vi "Lab Panel V6.00.vi"() -> ()   [LabVIEW 2017] (continued)
                  frame True {
                    n1786 = local read "DISP LAB05-1"() -> (w3328:T4)
                    n1787 = Unbundle(w3328) -> ("CYCLE"=w3336:dbl, "STATUS"=w3333:string)  [unwired: 1 out]
                    n1788 = global write "Global display 2.vi" "DISP LAB05-1"(w3328) -> ()
                    n1789 = Not Equal?(x=w3333, y="RUN") -> (x != y?=w3335:bool)
                    n1790 = local read "TDMS LAB05-1"() -> (w3339:refnum<k34>)
                    n1791 = Greater?(x=w3336, y=2.0) -> (0:w3337:bool)
                    n1792 = And(x=w3337, y=w3335) -> (x .and. y?=w3334:bool)
                    n1793 = case shown="True" w3334 {
                      tunnel: w3328 -> [_ w3347]
                      tunnel: w3339 -> [_ w3346]
                      tunnel: w3333 -> [_ w3345]
                      tunnel: w3332 -> [_ w3344]
                      tunnel: w3331 -> [_ w3343]
                      tunnel: w3330 -> [_ w3342]
                      tunnel: w3329 -> [_ w3341]
                      frame False {
                      }
                      frame True {
                        n1794 = stacked-sequence {
                          tunnel: w3347 -> [w3350 _ _]
                          tunnel: w3346 -> [_ w3352 _]
                          tunnel: w3345 -> [_ _ w3358]
                          tunnel: w3344 -> [_ _ w3357]
                          tunnel: w3343 -> [_ _ w3356]
                          tunnel: w3342 -> [_ _ w3355]
                          tunnel: w3341 -> [_ _ w3354]
                          frame #0 {
                            w3348 = FALSE
                            n1795 = local write "mail control"("END") -> ()
                            n1796 = Bundle(cluster=w3350) -> (w3351:T4)  [unwired: 3 in]
                            n1797 = local write "O/I  LAB05-1"(w3348) -> ()
                            n1798 = local write "RUN LAB05-1"(w3348) -> ()
                            n1799 = local write "run lab05-1"(w3348) -> ()
                            n1800 = local write "DISP LAB05-1"(w3351) -> ()
                          }
                          frame #1 {
                            n1801 = TDMS Close(11:w3352) -> (0:w3353:errorcluster)  [unwired: 1 in, 1 out]
                            n1802 = local write "data file error"(w3353) -> ()
                          }
                          frame #2 {
                            n1803 = stacked-sequence {
                              tunnel: "LAB05-1" -> [w3361 w3367]
                              tunnel: w3358 -> [_ w3366]
                              tunnel: w3357 -> [_ w3365]
                              tunnel: w3356 -> [_ w3364]
                              tunnel: w3355 -> [_ w3363]
                              tunnel: w3354 -> [_ w3362]
                              frame #0 {
                                n1804 = call "sub vi - defrag tdms v1.vi"("panel id"=w3361) -> ("error out"=w3360:errorcluster)  [unwired: 10 in]
                                n1805 = local write "data file error"(w3360) -> ()
                              }
                              frame #1 {
                                n1806 = Bundle("STATUS"=w3366, "OUT SERVER ADDRESS"=w3365, "FROM ACCOUNT"=w3364, "Mail Test File To:"=w3363, "Mail Test Fail"=w3362) -> (w3369:T30)  [unwired: 1 in]
                                n1807 = call "Save data file (pass-fail) v5.vi"("Input Cluster"=w3369, "panel id"=w3367) -> ("network file save error"=w3368:errorcluster)  [unwired: 8 in, 1 out]
                                n1808 = local write "data file error"(w3368) -> ()
                              }
                            }
                          }
                        }
                      }
                    }
                  }
                }
              }
              frame #9 {
                # "LAB05-2"
                n1809 = local read "run lab05-2"() -> (w3374:bool)
                n1810 = case shown="True" w3374 {
                  tunnel: w3373 -> [_ w3379]
                  tunnel: w3372 -> [_ w3378]
                  tunnel: w3371 -> [_ w3377]
                  tunnel: w3370 -> [_ w3376]
                  frame False {
                  }
                  frame True {
                    n1811 = local read "DISP LAB05-2"() -> (w3375:T4)
                    n1812 = Unbundle(w3375) -> ("CYCLE"=w3383:dbl, "STATUS"=w3380:string)  [unwired: 1 out]
                    n1813 = global write "Global display 2.vi" "DISP LAB05-2"(w3375) -> ()
                    n1814 = Not Equal?(x=w3380, y="RUN") -> (x != y?=w3382:bool)
                    n1815 = local read "TDMS LAB05-2"() -> (w3386:refnum<k34>)
                    n1816 = Greater?(x=w3383, y=2.0) -> (0:w3384:bool)
                    n1817 = And(x=w3384, y=w3382) -> (x .and. y?=w3381:bool)
                    n1818 = case shown="True" w3381 {
                      tunnel: w3375 -> [_ w3394]
                      tunnel: w3386 -> [_ w3393]
                      tunnel: w3380 -> [_ w3392]
                      tunnel: w3379 -> [_ w3391]
                      tunnel: w3378 -> [_ w3390]
                      tunnel: w3377 -> [_ w3389]
                      tunnel: w3376 -> [_ w3388]
                      frame False {
                      }
                      frame True {
                        n1819 = stacked-sequence {
                          tunnel: w3394 -> [w3397 _ _]
                          tunnel: w3393 -> [_ w3399 _]
                          tunnel: w3392 -> [_ _ w3405]
                          tunnel: w3391 -> [_ _ w3404]
                          tunnel: w3390 -> [_ _ w3403]
                          tunnel: w3389 -> [_ _ w3402]
                          tunnel: w3388 -> [_ _ w3401]
                          frame #0 {
                            w3395 = FALSE
                            n1820 = local write "mail control"("END") -> ()
                            n1821 = Bundle(cluster=w3397) -> (w3398:T4)  [unwired: 3 in]
                            n1822 = local write "RUN LAB05-2"(w3395) -> ()
                            n1823 = local write "O/I  LAB05-2"(w3395) -> ()
                            n1824 = local write "run lab05-2"(w3395) -> ()
                            n1825 = local write "DISP LAB05-2"(w3398) -> ()
                          }
                          frame #1 {
                            n1826 = TDMS Close(11:w3399) -> (0:w3400:errorcluster)  [unwired: 1 in, 1 out]
                            n1827 = local write "data file error"(w3400) -> ()
                          }
                          frame #2 {
                            n1828 = stacked-sequence {
                              tunnel: "LAB05-2" -> [w3408 w3414]
                              tunnel: w3405 -> [_ w3413]
                              tunnel: w3404 -> [_ w3412]
                              tunnel: w3403 -> [_ w3411]
                              tunnel: w3402 -> [_ w3410]
                              tunnel: w3401 -> [_ w3409]
                              frame #0 {
                                n1829 = call "sub vi - defrag tdms v1.vi"("panel id"=w3408) -> ("error out"=w3407:errorcluster)  [unwired: 10 in]
                                n1830 = local write "data file error"(w3407) -> ()
                              }
                              frame #1 {
                                n1831 = Bundle("STATUS"=w3413, "OUT SERVER ADDRESS"=w3412, "FROM ACCOUNT"=w3411, "Mail Test File To:"=w3410, "Mail Test Fail"=w3409) -> (w3416:T30)  [unwired: 1 in]
                                n1832 = call "Save data file (pass-fail) v5.vi"("Input Cluster"=w3416, "panel id"=w3414) -> ("network file save error"=w3415:errorcluster)  [unwired: 8 in, 1 out]
                                n1833 = local write "data file error"(w3415) -> ()
                              }
                            }
                          }
                        }
                      }
                    }
                  }
                }
              }
            }
            n1834 = global write "Global display 2.vi" "Mail test file to:"(w2923) -> ()
            n1835 = local read "Network Directory"() -> (w2929:path)
            n1836 = global write "Global 1.vi" "Network Drive"(w2929) -> ()
          }
          frame #8 {
            # "disable functions"
            n1837 = stacked-sequence {
              tunnel: w3426 -> [w3440 _ w3497]
              tunnel: w3425 -> [w3435 _ w3496]
              tunnel: w3424 -> [w3434 _ w3495]
              tunnel: w3423 -> [w3432 _ w3494]
              tunnel: w3422 -> [w3433 _ w3493]
              tunnel: w3421 -> [_ w3457 w3492]
              tunnel: w3420 -> [_ w3458 w3491]
              tunnel: w3419 -> [_ w3459 w3490]
              tunnel: w3418 -> [_ w3460 w3489]
              tunnel: w3417 -> [_ w3461 w3488]
              frame #0 {
                n1838 = Select(t=2, s=w3432, f=0) -> (s? t:f=w3428:i32)
                n1839 = Select(t=2, s=w3434, f=0) -> (s? t:f=w3429:i32)
                n1840 = Select(t=2, s=w3433, f=0) -> (s? t:f=w3427:i32)
                n1841 = Select(t=2, s=w3440, f=0) -> (s? t:f=w3431:i32)
                n1842 = Select(t=2, s=w3435, f=0) -> (s? t:f=w3430:i32)
                n1843 = property on="SELECT LAB02-2" class="RadioBtnsControl (strict)"("DisabledEnum"=w3428) -> ()  [unwired: 2 in, 2 out]
                n1844 = property on="SELECT LAB02-1" class="RadioBtnsControl (strict)"("DisabledEnum"=w3429) -> ()  [unwired: 2 in, 2 out]
                n1845 = property on="SELECT LAB03-1" class="RadioBtnsControl (strict)"("DisabledEnum"=w3427) -> ()  [unwired: 2 in, 2 out]
                n1846 = property on="SELECT LAB01-1" class="RadioBtnsControl (strict)"("DisabledEnum"=w3431) -> ()  [unwired: 2 in, 2 out]
                n1847 = property on="SELECT LAB01-2" class="RadioBtnsControl (strict)"("DisabledEnum"=w3430) -> ()  [unwired: 2 in, 2 out]
                n1848 = Not(x=w3440) -> (.not. x?=w3441:bool)
                n1849 = property on="RESULT LAB01-1" class="Bool (strict)"("Visible"=w3441) -> ()  [unwired: 2 in, 2 out]
                n1850 = Not(x=w3435) -> (.not. x?=w3439:bool)
                n1851 = Not(x=w3434) -> (.not. x?=w3438:bool)
                n1852 = Not(x=w3432) -> (.not. x?=w3437:bool)
                n1853 = property on="RESULT LAB01-2" class="Bool (strict)"("Visible"=w3439) -> ()  [unwired: 2 in, 2 out]
                n1854 = Not(x=w3433) -> (.not. x?=w3436:bool)
                n1855 = property on="RESULT LAB02-1" class="Bool (strict)"("Visible"=w3438) -> ()  [unwired: 2 in, 2 out]
                n1856 = property on="RESULT LAB02-2" class="Bool (strict)"("Visible"=w3437) -> ()  [unwired: 2 in, 2 out]
                n1857 = property on="RESULT LAB03-1" class="Bool (strict)"("Visible"=w3436) -> ()  [unwired: 2 in, 2 out]
                n1858 = property on="SET LAB01-1" class="Clust (strict)"("DisabledEnum"=w3431) -> ()  [unwired: 2 in, 2 out]
                n1859 = property on="SET LAB01-2" class="Clust (strict)"("DisabledEnum"=w3430) -> ()  [unwired: 2 in, 2 out]
                n1860 = property on="SET LAB02-1" class="Clust (strict)"("DisabledEnum"=w3429) -> ()  [unwired: 2 in, 2 out]
                n1861 = property on="SET LAB02-2" class="Clust (strict)"("DisabledEnum"=w3428) -> ()  [unwired: 2 in, 2 out]
                n1862 = property on="SET LAB03-1" class="Clust (strict)"("DisabledEnum"=w3427) -> ()  [unwired: 2 in, 2 out]
                n1863 = property on="O/I  LAB01-1" class="Bool (strict)"("DisabledEnum"=w3431) -> ()  [unwired: 2 in, 2 out]
                n1864 = property on="O/I  LAB01-2" class="Bool (strict)"("DisabledEnum"=w3430) -> ()  [unwired: 2 in, 2 out]
                n1865 = property on="O/I  LAB02-1" class="Bool (strict)"("DisabledEnum"=w3429) -> ()  [unwired: 2 in, 2 out]
                n1866 = property on="O/I  LAB02-2" class="Bool (strict)"("DisabledEnum"=w3428) -> ()  [unwired: 2 in, 2 out]
                n1867 = property on="O/I  LAB03-1" class="Bool (strict)"("DisabledEnum"=w3427) -> ()  [unwired: 2 in, 2 out]
              }
              frame #1 {
                n1868 = Select(t=2, s=w3461, f=0) -> (s? t:f=w3452:i32)
                n1869 = Select(t=2, s=w3460, f=0) -> (s? t:f=w3453:i32)
                n1870 = Select(t=2, s=w3457, f=0) -> (s? t:f=w3456:i32)
                n1871 = Select(t=2, s=w3458, f=0) -> (s? t:f=w3455:i32)
                n1872 = Select(t=2, s=w3459, f=0) -> (s? t:f=w3454:i32)
                n1873 = property on="SELECT LAB05-2" class="RadioBtnsControl (strict)"("DisabledEnum"=w3452) -> ()  [unwired: 2 in, 2 out]
                n1874 = property on="SELECT LAB05-1" class="RadioBtnsControl (strict)"("DisabledEnum"=w3453) -> ()  [unwired: 2 in, 2 out]
                n1875 = property on="SELECT LAB03-2" class="RadioBtnsControl (strict)"("DisabledEnum"=w3456) -> ()  [unwired: 2 in, 2 out]
                n1876 = property on="SELECT LAB04-1" class="RadioBtnsControl (strict)"("DisabledEnum"=w3455) -> ()  [unwired: 2 in, 2 out]
                n1877 = property on="SELECT LAB04-2" class="RadioBtnsControl (strict)"("DisabledEnum"=w3454) -> ()  [unwired: 2 in, 2 out]
                n1878 = property on="SET LAB05-2" class="Clust (strict)"("DisabledEnum"=w3452) -> ()  [unwired: 2 in, 2 out]
                n1879 = property on="SET LAB05-1" class="Clust (strict)"("DisabledEnum"=w3453) -> ()  [unwired: 2 in, 2 out]
                n1880 = property on="SET LAB03-2" class="Clust (strict)"("DisabledEnum"=w3456) -> ()  [unwired: 2 in, 2 out]
                n1881 = property on="SET LAB04-1" class="Clust (strict)"("DisabledEnum"=w3455) -> ()  [unwired: 2 in, 2 out]
                n1882 = property on="SET LAB04-2" class="Clust (strict)"("DisabledEnum"=w3454) -> ()  [unwired: 2 in, 2 out]
                n1883 = property on="O/I  LAB05-2" class="Bool (strict)"("DisabledEnum"=w3452) -> ()  [unwired: 2 in, 2 out]
                n1884 = property on="O/I  LAB05-1" class="Bool (strict)"("DisabledEnum"=w3453) -> ()  [unwired: 2 in, 2 out]
                n1885 = property on="O/I  LAB04-1" class="Bool (strict)"("DisabledEnum"=w3455) -> ()  [unwired: 2 in, 2 out]
                n1886 = property on="O/I  LAB04-2" class="Bool (strict)"("DisabledEnum"=w3454) -> ()  [unwired: 2 in, 2 out]
                n1887 = property on="O/I  LAB03-2" class="Bool (strict)"("DisabledEnum"=w3456) -> ()  [unwired: 2 in, 2 out]
                n1888 = Not(x=w3461) -> (.not. x?=w3462:bool)
                n1889 = Not(x=w3460) -> (.not. x?=w3463:bool)
                n1890 = Not(x=w3459) -> (.not. x?=w3464:bool)
                n1891 = property on="RESULT LAB05-2" class="Bool (strict)"("Visible"=w3462) -> ()  [unwired: 2 in, 2 out]
                n1892 = property on="RESULT LAB05-1" class="Bool (strict)"("Visible"=w3463) -> ()  [unwired: 2 in, 2 out]
                n1893 = Not(x=w3458) -> (.not. x?=w3465:bool)
                n1894 = property on="RESULT LAB04-2" class="Bool (strict)"("Visible"=w3464) -> ()  [unwired: 2 in, 2 out]
                n1895 = Not(x=w3457) -> (.not. x?=w3466:bool)
                n1896 = property on="RESULT LAB04-1" class="Bool (strict)"("Visible"=w3465) -> ()  [unwired: 2 in, 2 out]
                n1897 = property on="RESULT LAB03-2" class="Bool (strict)"("Visible"=w3466) -> ()  [unwired: 2 in, 2 out]
              }
              frame #2 {
                # "disable calibrate if any test running"
                n1898 = Or(x=w3489, y=w3488) -> (x .or. y?=w3482:bool)
                n1899 = Or(x=w3491, y=w3490) -> (x .or. y?=w3484:bool)
                n1900 = Or(x=w3495, y=w3494) -> (x .or. y?=w3486:bool)
                n1901 = Or(x=w3493, y=w3492) -> (x .or. y?=w3485:bool)
                n1902 = Or(x=w3497, y=w3496) -> (x .or. y?=w3487:bool)
                n1903 = Or(x=w3485, y=w3484) -> (x .or. y?=w3483:bool)
                n1904 = Or(x=w3487, y=w3486) -> (x .or. y?=w3481:bool)
                n1905 = Or(x=w3483, y=w3482) -> (x .or. y?=w3480:bool)
                n1906 = Or(x=w3481, y=w3480) -> (x .or. y?=w3477:bool)
                "Any Test Running" <- w3477
                n1907 = case shown="False" w3477 {
                  tunnel: [0 2] -> w3479
                  frame False {
                  }
                  frame True {
                  }
                }
                n1908 = property on="JIG TEST" class="Clust (strict)"("DisabledEnum"=w3479) -> ()  [unwired: 2 in, 2 out]
                n1909 = property on="Network Directory" class="Path"("DisabledEnum"=w3479) -> ()  [unwired: 2 in, 2 out]
                n1910 = property on="MAIL SETTINGS" class="Clust (strict)"("DisabledEnum"=w3479) -> ()  [unwired: 2 in, 2 out]
                n1911 = property on="SET (cal)" class="Bool (strict)"("DisabledEnum"=w3479) -> ()  [unwired: 2 in, 2 out]
                n1912 = property on="ADMIN" class="Bool (strict)"("DisabledEnum"=0) -> ()  [unwired: 2 in, 2 out]
              }
            }
          }
          frame #9 {
            # "Note : JIG LAB0X-N   are written to digital I/O in frame 11"
            # "Drive jigs"
            n1913 = stacked-sequence {
              frame #0 {
                # "jig on"
                n1914 = local read "jig cycle"() -> (w3505:dbl)
                n1915 = property on="JIG TEST" class="Clust (strict)"() -> ("DisabledEnum"=w3502:T17)  [unwired: 2 in, 2 out]
                n1916 = Equal?(x=w3502, y=2) -> (x = y?=w3501:bool)
                n1917 = Equal?(x=w3505, y=0) -> (x = y?=w3503:bool)
                n1918 = And(x=w3503, y=w3501) -> (x .and. y?=w3500:bool)
                n1919 = case shown="True" w3500 {
                  frame False {
                  }
                  frame True {
                    n1920 = local read "run lab01-2"() -> (w3515:bool)
                    n1921 = local read "run lab01-1"() -> (w3516:bool)
                    n1922 = local read "run lab02-1"() -> (w3514:bool)
                    n1923 = local read "run lab02-2"() -> (w3513:bool)
                    n1924 = local read "run lab03-1"() -> (w3512:bool)
                    n1925 = local read "run lab03-2"() -> (w3511:bool)
                    n1926 = local read "run lab04-1"() -> (w3510:bool)
                    n1927 = local read "run lab04-2"() -> (w3509:bool)
                    n1928 = local read "run lab05-1"() -> (w3508:bool)
                    n1929 = local read "run lab05-2"() -> (w3507:bool)
                    n1930 = local write "JIG LAB01-2"(w3515) -> ()
                    n1931 = local write "JIG LAB03-2"(w3511) -> ()
                    n1932 = local write "JIG LAB01-1"(w3516) -> ()
                    n1933 = local write "JIG LAB02-1"(w3514) -> ()
                    n1934 = local write "JIG LAB02-2"(w3513) -> ()
                    n1935 = local write "JIG LAB03-1"(w3512) -> ()
                    n1936 = local write "JIG LAB04-1"(w3510) -> ()
                    n1937 = local write "JIG LAB04-2"(w3509) -> ()
                    n1938 = local write "JIG LAB05-1"(w3508) -> ()
                    n1939 = local write "JIG LAB05-2"(w3507) -> ()
                  }
                }
              }
              frame #1 {
                # "jig off"
                n1940 = local read "jig cycle"() -> (w3523:dbl)
                n1941 = local read "on loops"() -> (w3522:dbl)
                n1942 = property on="JIG TEST" class="Clust (strict)"() -> ("DisabledEnum"=w3521:T17)  [unwired: 2 in, 2 out]
                n1943 = Equal?(x=w3521, y=2) -> (x = y?=w3519:bool)
                n1944 = Equal?(x=w3523, y=w3522) -> (x = y?=w3518:bool)
                n1945 = And(x=w3518, y=w3519) -> (x .and. y?=w3517:bool)
                n1946 = case shown="True" w3517 {
                  frame False {
                  }
                  frame True {
                    w3574 = FALSE
                    w3575 = TRUE
                    w3573 = 2
                    n1947 = local read "SELECT LAB05-2"() -> (w3564:T3)
                    n1948 = local read "SELECT LAB04-2"() -> (w3566:T3)
                    n1949 = local read "SELECT LAB04-1"() -> (w3567:T3)
                    n1950 = local read "SELECT LAB05-1"() -> (w3565:T3)
                    n1951 = local read "SELECT LAB03-2"() -> (w3568:T3)
                    n1952 = local read "SELECT LAB02-1"() -> (w3571:T3)
                    n1953 = local read "SELECT LAB03-1"() -> (w3569:T3)
                    n1954 = local read "SELECT LAB02-2"() -> (w3570:T3)
                    n1955 = local read "SELECT LAB01-2"() -> (w3572:T3)
                    n1956 = local read "run lab05-1"() -> (w3534:bool)
                    n1957 = local read "run lab05-2"() -> (w3533:bool)
                    n1958 = local read "run lab04-2"() -> (w3535:bool)
                    n1959 = local read "SELECT LAB01-1"() -> (w3576:T3)
                    n1960 = local read "run lab04-1"() -> (w3536:bool)
                    n1961 = local read "run lab01-1"() -> (w3552:bool)
                    n1962 = local read "run lab01-2"() -> (w3541:bool)
                    n1963 = local read "run lab03-2"() -> (w3537:bool)
                    n1964 = local read "run lab03-1"() -> (w3538:bool)
                    n1965 = local read "run lab02-1"() -> (w3540:bool)
                    n1966 = local read "run lab02-2"() -> (w3539:bool)
                    n1967 = Equal?(x=w3573, y=w3569) -> (x = y?=w3547:bool)
                    n1968 = Equal?(x=w3573, y=w3568) -> (x = y?=w3546:bool)
                    n1969 = Equal?(x=w3573, y=w3567) -> (x = y?=w3545:bool)
                    n1970 = Equal?(x=w3573, y=w3566) -> (x = y?=w3544:bool)
                    n1971 = Equal?(x=w3573, y=w3565) -> (x = y?=w3543:bool)
                    n1972 = Equal?(x=w3573, y=w3564) -> (x = y?=w3542:bool)
                    n1973 = Equal?(x=w3573, y=w3576) -> (x = y?=w3553:bool)
                    n1974 = Equal?(x=w3573, y=w3571) -> (x = y?=w3549:bool)
                    n1975 = Equal?(x=w3573, y=w3570) -> (x = y?=w3548:bool)
                    n1976 = Equal?(x=w3573, y=w3572) -> (x = y?=w3550:bool)
                    n1977 = And(x=w3544, y=w3535) -> (x .and. y?=w3526:bool)
                    n1978 = And(x=w3547, y=w3538) -> (x .and. y?=w3529:bool)
                    n1979 = And(x=w3545, y=w3536) -> (x .and. y?=w3527:bool)
                    n1980 = And(x=w3542, y=w3533) -> (x .and. y?=w3524:bool)
                    n1981 = And(x=w3548, y=w3539) -> (x .and. y?=w3530:bool)
                    n1982 = And(x=w3546, y=w3537) -> (x .and. y?=w3528:bool)
                    n1983 = And(x=w3543, y=w3534) -> (x .and. y?=w3525:bool)
                    n1984 = And(x=w3550, y=w3541) -> (x .and. y?=w3532:bool)
                    n1985 = And(x=w3553, y=w3552) -> (x .and. y?=w3551:bool)
                    n1986 = And(x=w3549, y=w3540) -> (x .and. y?=w3531:bool)
                    n1987 = Select(t=w3575, s=w3551, f=w3574) -> (s? t:f=w3554:bool)
                    n1988 = Select(t=w3575, s=w3532, f=w3574) -> (s? t:f=w3555:bool)
                    n1989 = Select(t=w3575, s=w3531, f=w3574) -> (s? t:f=w3556:bool)
                    n1990 = Select(t=w3575, s=w3530, f=w3574) -> (s? t:f=w3557:bool)
                    n1991 = Select(t=w3575, s=w3529, f=w3574) -> (s? t:f=w3558:bool)
                    n1992 = Select(t=w3575, s=w3528, f=w3574) -> (s? t:f=w3559:bool)
                    n1993 = Select(t=w3575, s=w3527, f=w3574) -> (s? t:f=w3560:bool)
                    n1994 = Select(t=w3575, s=w3526, f=w3574) -> (s? t:f=w3561:bool)
                    n1995 = Select(t=w3575, s=w3525, f=w3574) -> (s? t:f=w3562:bool)
                    n1996 = Select(t=w3575, s=w3524, f=w3574) -> (s? t:f=w3563:bool)
                    n1997 = local write "JIG LAB03-2"(w3559) -> ()
                    n1998 = local write "JIG LAB02-1"(w3556) -> ()
                    n1999 = local write "JIG LAB02-2"(w3557) -> ()
                    n2000 = local write "JIG LAB01-2"(w3555) -> ()
                    n2001 = local write "JIG LAB03-1"(w3558) -> ()
                    n2002 = local write "JIG LAB01-1"(w3554) -> ()
                    n2003 = local write "JIG LAB05-2"(w3563) -> ()
                    n2004 = local write "JIG LAB04-1"(w3560) -> ()
                    n2005 = local write "JIG LAB05-1"(w3562) -> ()
                    n2006 = local write "JIG LAB04-2"(w3561) -> ()
                  }
                }
              }
            }
          }
          frame #10 {
            # "Note : JIG LAB0X-N   are written to digital I/O in frame 11"
            # "enable  jig test output if no test busy"
            n2007 = property on="JIG TEST" class="Clust (strict)"() -> ("DisabledEnum"=w3579:T17)  [unwired: 2 in, 2 out]
            n2008 = Equal?(x=w3579, y=0) -> (x = y?=w3577:bool)
            n2009 = case shown="True" w3577 {
              frame False {
              }
              frame True {
                n2010 = local read "JIG TEST"() -> (w3590:T11)
                n2011 = Unbundle(w3590) -> ("LAB01-1"=w3589:bool, "LAB01-2"=w3588:bool, "LAB02-1"=w3587:bool, "LAB02-2"=w3586:bool, "LAB03-1"=w3585:bool, "LAB03-2"=w3584:bool, "LAB04-1"=w3583:bool, "LAB04-2"=w3582:bool, "LAB05-1"=w3581:bool, "LAB05-2"=w3580:bool)
                n2012 = local write "JIG LAB05-1"(w3581) -> ()
                n2013 = local write "JIG LAB05-2"(w3580) -> ()
                n2014 = local write "JIG LAB04-1"(w3583) -> ()
                n2015 = local write "JIG LAB04-2"(w3582) -> ()
                n2016 = local write "JIG LAB03-2"(w3584) -> ()
                n2017 = local write "JIG LAB01-1"(w3589) -> ()
                n2018 = local write "JIG LAB02-1"(w3587) -> ()
                n2019 = local write "JIG LAB03-1"(w3585) -> ()
                n2020 = local write "JIG LAB01-2"(w3588) -> ()
                n2021 = local write "JIG LAB02-2"(w3586) -> ()
              }
            }
          }
          frame #11 {
            w3592 = FALSE
            # "Drive digital output and RESET  USB and temperature network if required."
            n2022 = global read "Global display 3.vi" "cycle O/F"() -> (w3601:bool)
            n2023 = case shown="False" w3601 {
              tunnel: [w3740 FALSE] -> w3600
              frame False {
                n2024 = local read "Analog error"() -> (w3742:bool)
                n2025 = local read "Reset Measuring"() -> (w3741:bool)
                n2026 = Or(x=w3741, y=w3742) -> (x .or. y?=w3740:bool)
              }
              frame True {
              }
            }
            n2027 = local read "O/I  LAB01-1"() -> (w3620:bool)
            n2028 = local read "JIG LAB01-1"() -> (w3619:bool)
            n2029 = local read "O/I  LAB01-2"() -> (w3618:bool)
            n2030 = local read "JIG LAB01-2"() -> (w3617:bool)
            n2031 = local read "O/I  LAB02-1"() -> (w3616:bool)
            n2032 = local read "JIG LAB02-1"() -> (w3615:bool)
            n2033 = local read "O/I  LAB02-2"() -> (w3614:bool)
            n2034 = local read "JIG LAB02-2"() -> (w3613:bool)
            n2035 = local read "O/I  LAB03-1"() -> (w3612:bool)
            n2036 = local read "JIG LAB03-1"() -> (w3611:bool)
            n2037 = local read "O/I  LAB03-2"() -> (w3610:bool)
            n2038 = local read "JIG LAB03-2"() -> (w3609:bool)
            n2039 = local read "O/I  LAB04-1"() -> (w3608:bool)
            n2040 = local read "JIG LAB04-1"() -> (w3607:bool)
            n2041 = local read "O/I  LAB04-2"() -> (w3598:bool)
            n2042 = local read "JIG LAB04-2"() -> (w3597:bool)
            n2043 = local read "O/I  LAB05-1"() -> (w3596:bool)
            n2044 = local read "JIG LAB05-1"() -> (w3595:bool)
            n2045 = local read "O/I  LAB05-2"() -> (w3594:bool)
            n2046 = local read "JIG LAB05-2"() -> (w3593:bool)
            n2047 = Build Array(w3613, w3612, w3611, w3610, w3609, w3608, w3607) -> (w3605:bool[])
            "USB OUT 1" <- w3605
            n2048 = Build Array(w3620, w3619, w3618, w3617, w3616, w3615, w3614) -> (w3606:bool[])
            "USB OUT 0" <- w3606
            n2049 = Build Array(w3598, w3597, w3596, w3595, w3594, w3593, w3592, w3592) -> (w3604:bool[])
            "USB OUT 2" <- w3604
            n2050 = Not(x=w3601) -> (.not. x?=w3602:bool)
            n2051 = local read "DAQ Simulate"() -> (w3603:bool)
            n2052 = And(x=w3602, y=w3600) -> (x .and. y?=w3599:bool)
            n2053 = stacked-sequence {
              tunnel: w3606 -> [w3624 w3631]
              tunnel: w3605 -> [w3623 w3630]
              tunnel: w3604 -> [w3622 w3629]
              tunnel: w3603 -> [w3621 w3632]
              tunnel: w3599 -> [_ w3633]
              tunnel: w3591 -> [_ w3628]
              frame #0 {
                # "drive outputs for normal use"
                n2054 = case shown="False" w3621 {
                  tunnel: w3624 -> [w3627 _]
                  tunnel: w3623 -> [w3626 _]
                  tunnel: w3622 -> [w3625 _]
                  frame False {
                    n2055 = call "sub vi - Drive Relays All v6.vi"("Array #2"=w3625, "Array #1"=w3626, "Array #0"=w3627) -> ()  [unwired: 8 in, 1 out]
                  }
                  frame True {
                  }
                }
              }
              frame #1 {
                # "USB  reset routine"
                n2056 = case shown="True" w3633 {
                  tunnel: w3632 -> [_ w3638]
                  tunnel: w3631 -> [_ w3637]
                  tunnel: w3630 -> [_ w3636]
                  tunnel: w3629 -> [_ w3635]
                  tunnel: w3628 -> [_ w3634]
                  frame False {
                  }
                  frame True {
                    n2057 = stacked-sequence {
                      seq-local: [w3640 _ _ _ _] -> [_ w3647 _ _ _]
                      tunnel: w3638 -> [_ w3651 _ _ _]
                      tunnel: w3637 -> [_ w3650 _ _ _]
                      tunnel: w3636 -> [_ w3649 _ _ _]
                      tunnel: w3635 -> [_ w3648 _ _ _]
                      tunnel: w3634 -> [_ w3646 _ _ _]
                      frame #0 {
                        n2058 = case shown="False" "Auto Reset" {
                          tunnel: [w3643 FALSE] -> w3641
                          frame False {
                            n2059 = Two Button Dialog(message="System reset") -> (T button?=w3643:bool)  [unwired: 2 in]
                          }
                          frame True {
                          }
                        }
                        n2060 = disable-structure shown="Disabled" {
                          frame Disabled {
                            n2061 = local write "Tab Control 2"(5) -> ()
                          }
                          frame Enabled {
                          }
                        }
                        n2062 = Or(x="Auto Reset", y=w3641) -> (x .or. y?=w3640:bool)
                      }
                      frame #1 {
                        n2063 = case shown="True" w3647 {
                          tunnel: w3651 -> [_ w3658]
                          tunnel: w3650 -> [_ w3657]
                          tunnel: w3649 -> [_ w3656]
                          tunnel: w3648 -> [_ w3655]
                          tunnel: w3646 -> [_ w3652]
                          frame False {
                          }
                          frame True {
                            n2064 = stacked-sequence {
                              tunnel: w3658 -> [_ w3677 _]
                              tunnel: bool[] [] -> [w3661 w3676 w3697]
                              tunnel: w3657 -> [_ _ w3696]
                              tunnel: w3656 -> [w3660 _ w3695]
                              tunnel: w3655 -> [w3659 _ w3694]
                              tunnel: 5000 -> [w3662 _ w3693]
                              tunnel: w3652 -> [_ w3675 _]
                              frame #0 {
                                # "switch off test stations for system reset"
                                n2065 = stacked-sequence {
                                tunnel: w3662 -> [w3666 w3670 w3672]
                                tunnel: w3661 -> [w3665 w3669 w3673]
                                tunnel: w3660 -> [w3664 _ _]
                                tunnel: w3659 -> [w3663 w3668 _]
                                frame #0 {
                                # "drive 1st 7 inputs"
                                n2066 = call "sub vi - Drive Relays All v6.vi"("Array #2"=w3663, "Array #1"=w3664, "Array #0"=w3665) -> ()  [unwired: 8 in, 1 out]
                                n2067 = call "Message Display V1.vi"("Message"="Delay off LAB 01-1 to 02-1", "Delay mS"=w3666) -> ()  [unwired: 10 in]
                                }
                                frame #1 {
                                # "drive 2nd 7 inputs"
                                n2068 = call "sub vi - Drive Relays All v6.vi"("Array #2"=w3668, "Array #1"=w3669, "Array #0"=w3669) -> ()  [unwired: 8 in, 1 out]
                                n2069 = call "Message Display V1.vi"("Message"="Delay off LAB 02-2 to 04-1", "Delay mS"=w3670) -> ()  [unwired: 10 in]
                                }
                                frame #2 {
                                # "drive 3rd 7 inputs"
                                n2070 = call "sub vi - Drive Relays All v6.vi"("Array #2"=w3673, "Array #1"=w3673, "Array #0"=w3673) -> ()  [unwired: 8 in, 1 out]
                                n2071 = call "Message Display V1.vi"("Message"="Delay off LAB 04-2 to 05-2", "Delay mS"=w3672) -> ()  [unwired: 10 in]
                                }
                                }
                              }
                              frame #1 {
                                # "reset all usb modules"
                                n2072 = stacked-sequence {
                                tunnel: w3677 -> [_ w3683]
                                tunnel: w3676 -> [w3680 _]
                                tunnel: w3675 -> [_ w3681]
                                frame #0 {
                                n2073 = local write "AI Task"(FALSE) -> ()
                                n2074 = call "sub vi - Drive Relays All v6.vi"("Array #2"=bool[] [FALSE, FALSE, FALSE, FALSE, FALSE, FALSE, TRUE, FALSE], "Array #1"=w3680, "Array #0"=w3680) -> ()  [unwired: 8 in, 1 out]
                                }
                                frame #1 {
                                n2075 = call "Reset Meas v 5.vi"("simulate"=w3683) -> ("Reset Error"=w3682:bool)  [unwired: 10 in]
                                n2076 = case shown="True" w3682 {
                                tunnel: w3681 -> [_ w3685]
                                frame False {
                                "Reset Error" <- FALSE
                                }
                                frame True {
                                n2077 = local read "RATE (Hz)"() -> (w3689:dbl)
                                n2078 = local read "SAMPLES"() -> (w3688:dbl)
                                n2079 = call "sub vi - AI USB4704 (3)  Create Task v4.vi"("Test"=w3685, "Rate Hz"=w3689, "Samples"=w3688) -> ("TASK USB 0"=w3692:i32, "TASK USB 1"=w3691:i32, "TASK USB 2"=w3690:i32, "AI Task Er"=w3686:bool)  [unwired: 5 in, 4 out]
                                n2080 = local write "AI Task"(TRUE) -> ()
                                n2081 = local write "Reset Error"(w3686) -> ()
                                n2082 = local write "AI Task2"(w3690) -> ()
                                n2083 = local write "AI Task1"(w3691) -> ()
                                n2084 = local write "AI Task0"(w3692) -> ()
                                }
                                }
                                }
                                }
                              }
                              frame #2 {
                                # "switch test stations back on after reset"
                                n2085 = stacked-sequence {
                                tunnel: w3697 -> [w3701 w3704 _]
                                tunnel: w3696 -> [w3700 w3706 w3711]
                                tunnel: w3693 -> [w3699 w3702 w3708]
                                tunnel: w3695 -> [_ w3705 w3710]
                                tunnel: w3694 -> [_ _ w3707]
                                frame #0 {
                                # "drive 1st 7 inputs"
                                n2086 = call "sub vi - Drive Relays All v6.vi"("Array #2"=w3701, "Array #1"=w3701, "Array #0"=w3700) -> ()  [unwired: 8 in, 1 out]
                                n2087 = call "Message Display V1.vi"("Message"="Delay on LAB 01-1 to 02-1", "Delay mS"=w3699) -> ()  [unwired: 10 in]
                                }
                                frame #1 {
                                # "drive 1st & 2nd outputs"
                                n2088 = call "sub vi - Drive Relays All v6.vi"("Array #2"=w3704, "Array #1"=w3705, "Array #0"=w3706) -> ()  [unwired: 8 in, 1 out]
                                n2089 = call "Message Display V1.vi"("Message"="Delay on LAB 02-2 to 04-1", "Delay mS"=w3702) -> ()  [unwired: 10 in]
                                }
                                frame #2 {
                                n2090 = call "sub vi - Drive Relays All v6.vi"("Array #2"=w3707, "Array #1"=w3710, "Array #0"=w3711) -> ()  [unwired: 8 in, 1 out]
                                n2091 = call "Message Display V1.vi"("Message"="Delay on LAB 04-2 to 05-2", "Delay mS"=w3708) -> ()  [unwired: 10 in]
                                }
                                }
                              }
                            }
                          }
                        }
                      }
                      frame #2 {
                        w3712 = 0
                        w3713 = FALSE
                        # "set all back to zero"
                        n2092 = local read "Total USB resets"() -> (w3715:dbl)
                        n2093 = local read "Resets Done"() -> (w3717:dbl)
                        n2094 = local write "Reset Measuring"(w3713) -> ()
                        n2095 = local write "Analog error"(w3713) -> ()
                        n2096 = local write "Er USB#2"(w3712) -> ()
                        n2097 = local write "Er USB#0"(w3712) -> ()
                        n2098 = local write "Er USB#1"(w3712) -> ()
                        n2099 = local write "Error USB #0"(w3713) -> ()
                        n2100 = local write "Error USB #1"(w3713) -> ()
                        n2101 = local write "Error USB #2"(w3713) -> ()
                        n2102 = Increment(x=w3715) -> (x+1=w3714:dbl)
                        n2103 = Increment(x=w3717) -> (x+1=→"Resets Done":dbl)
                        n2104 = local write "Total USB resets"(w3714) -> ()
                      }
                      frame #3 {
                        # "save reset value"
                        n2105 = String To Path(string="c:\\crabtree\\Set Up\\") -> (path=w3727:path)
                        n2106 = Build Path(base path=w3727, name or relative path="USB resets.bin") -> (appended path=w3720:path)
                        n2107 = Create Folder(path (use dialog)=w3727) -> (error out=w3719:errorcluster)  [unwired: 2 in, 2 out]
                        n2108 = local read "Total USB resets"() -> (w3718:dbl)
                        n2109 = call <vilib>:"Clear Errors.vi"("error in (no error)"=w3719) -> ()  [unwired: 5 in, 2 out]
                        n2110 = Open/Create/Replace File(file path (use dialog)=w3720, operation (0:open)=T18."replace or create") -> (refnum out=w3725:refnum<file>, error out=w3724:errorcluster)  [unwired: 4 in, 1 out]
                        n2111 = Write to Binary File(file (use dialog)=w3725, data=w3718, error in=w3724) -> (refnum out=w3723:refnum<file>, error out=w3722:errorcluster)  [unwired: 3 in, 1 out]
                        n2112 = Close File(refnum=w3723, error in=w3722) -> (error out=w3721:errorcluster)  [unwired: 1 out]
                        n2113 = local write "data file error"(w3721) -> ()
                      }
                      frame #4 {
                        # "mail reset value"
                        n2114 = local read "MAIL SETTINGS"() -> (w3733:T8)
                        n2115 = local read "Total USB resets"() -> (w3737:dbl)
                        n2116 = Unbundle(w3733) -> ("OUT SERVER ADDRESS"=w3739:string, "FROM ACCOUNT"=w3738:string)  [unwired: 5 out]
                        n2117 = Number To Decimal String(number=w3737) -> (decimal integer string=w3735:string)  [unwired: 1 in]
                        n2118 = Concatenate Strings("Total USB resets: ", w3735) -> (w3734:string)
                        n2119 = call "Lab Send Mail Test.vi"("TO:"="mikewestwood@gmail.com", "subject"=w3734, "from"=w3738, "out going server"=w3739) -> ("error out"=w3732:errorcluster)  [unwired: 11 in]
                        n2120 = Bundle(cluster=w3733, "mail error"=w3732) -> (w3731:T8)  [unwired: 6 in]
                        n2121 = local write "MAIL SETTINGS"(w3731) -> ()
                      }
                    }
                  }
                }
              }
            }
          }
          frame #12 {
            # "if all test panels are off stop analog read"
            n2122 = local read "O/I  LAB03-1"() -> (w3766:bool)
            n2123 = local read "O/I  LAB03-2"() -> (w3765:bool)
            n2124 = local read "O/I  LAB04-1"() -> (w3764:bool)
            n2125 = local read "O/I  LAB04-2"() -> (w3763:bool)
            n2126 = local read "O/I  LAB05-1"() -> (w3762:bool)
            n2127 = local read "O/I  LAB05-2"() -> (w3761:bool)
            n2128 = local read "O/I  LAB02-2"() -> (w3767:bool)
            n2129 = local read "O/I  LAB02-1"() -> (w3768:bool)
            n2130 = local read "O/I  LAB01-2"() -> (w3769:bool)
            n2131 = local read "O/I  LAB01-1"() -> (w3770:bool)
            n2132 = Or(x=w3762, y=w3761) -> (x .or. y?=w3759:bool)
            n2133 = Or(x=w3764, y=w3763) -> (x .or. y?=w3760:bool)
            n2134 = Or(x=w3768, y=w3767) -> (x .or. y?=w3758:bool)
            n2135 = Or(x=w3766, y=w3765) -> (x .or. y?=w3756:bool)
            n2136 = Or(x=w3770, y=w3769) -> (x .or. y?=w3757:bool)
            n2137 = Or(x=w3760, y=w3759) -> (x .or. y?=w3753:bool)
            n2138 = Or(x=w3757, y=w3758) -> (x .or. y?=w3755:bool)
            n2139 = Or(x=w3755, y=w3756) -> (x .or. y?=w3754:bool)
            n2140 = Or(x=w3754, y=w3753) -> (x .or. y?=w3751:bool)
            n2141 = local read "Any Test Running"() -> (w3752:bool)
            n2142 = local read "AI Task"() -> (w3747:bool)
            n2143 = Or(x=w3751, y=w3752) -> (x .or. y?=w3746:bool)
            n2144 = Not(x=w3746) -> (.not. x?=w3750:bool)
            n2145 = And(x=w3750, y=w3747) -> (x .and. y?=w3749:bool)
            n2146 = Not(x=w3747) -> (.not. x?=w3748:bool)
            n2147 = And(x=w3746, y=w3748) -> (x .and. y?=w3745:bool)
            n2148 = case shown="True" w3749 {
              frame False {
              }
              frame True {
                # "close task if no test"
                n2149 = local write "AI Task"(FALSE) -> ()
                n2150 = call "sub vi - AI USB4704 (3)  Close Task v2.vi"() -> ()  [unwired: 16 in]
              }
            }
            n2151 = case shown="True" w3745 {
              tunnel: w3744 -> [_ w3771]
              frame False {
              }
              frame True {
                # "create task for test"
                n2152 = local read "SAMPLES"() -> (w3773:dbl)
                n2153 = local read "RATE (Hz)"() -> (w3772:dbl)
                n2154 = call "sub vi - AI USB4704 (3)  Create Task v4.vi"("Test"=w3771, "Rate Hz"=w3772, "Samples"=w3773) -> ("TASK USB 0"=w3774:i32, "TASK USB 1"=w3775:i32, "TASK USB 2"=w3776:i32)  [unwired: 5 in, 5 out]
                n2155 = local write "AI Task0"(w3774) -> ()
                n2156 = local write "AI Task1"(w3775) -> ()
                n2157 = local write "AI Task2"(w3776) -> ()
                n2158 = local write "AI Task"(TRUE) -> ()
              }
            }
          }
          frame #13 {
            # "get all analog values from USB devices"
            n2159 = local read "on loops"() -> (w3790:dbl)
            n2160 = local read "jig cycle"() -> (w3787:dbl)
            n2161 = Add(x=w3790, y=3) -> (x+y=w3788:dbl)
            n2162 = Equal?(x=w3787, y=3) -> (x = y?=w3785:bool)
            n2163 = Equal?(x=w3787, y=w3788) -> (x = y?=w3786:bool)
            n2164 = Or(x=w3785, y=w3786) -> (x .or. y?=w3784:bool)
            "Process AIs" <- w3784
            n2165 = global write "Global display 3.vi" "cycle O/F"(w3785) -> ()
            n2166 = call "Check for valid PF.vi"("Min V"="Min V", "Init"=TRUE, "Min I"="Min I") -> ("PF Out"=w3779:dbl)  [unwired: 6 in, 2 out]
            n2167 = case shown="True" w3784 {
              tunnel: w3785 -> [_ w3796]
              tunnel: w3783 -> [_ w3793]
              tunnel: w3779 -> [_ _]
              frame False {
              }
              frame True {
                n2168 = local read "DAQ Simulate"() -> (w3799:bool)
                n2169 = case shown="False" w3799 {
                  tunnel: [w3815 dynamicdata[] [] ("array GRAPH")] -> w3805
                  tunnel: [w3814 w3840] -> w3804
                  tunnel: [w3813 w3840] -> w3803
                  tunnel: [w3812 w3840] -> w3802
                  tunnel: [w3811 w3840] -> w3801
                  tunnel: [w3810 w3840] -> w3800
                  tunnel: w3796 -> [_ w3844]
                  tunnel: [w3809 "Ambient Volts"] -> w3795
                  tunnel: [w3808 bool[] []] -> w3794
                  tunnel: w3793 -> [w3807 _]
                  tunnel: [w3806 0.3 ("Analog loop time")] -> w3792
                  frame False {
                    # "analog in"
                    n2170 = case shown="True" w3807 {
                      tunnel: [dynamicdata[] [] ("array GRAPH") w3834] -> w3815
                      tunnel: [w3817 w3833] -> w3814
                      tunnel: [w3817 w3832] -> w3813
                      tunnel: [w3817 w3831] -> w3812
                      tunnel: [w3817 w3830] -> w3811
                      tunnel: [w3817 w3829] -> w3810
                      tunnel: [3 w3828] -> w3809
                      tunnel: [bool[] [] w3827] -> w3808
                      tunnel: [0.0 w3823] -> w3806
                      frame False {
                        w3818 = 0.0
                        # "no test"
                        n2171 = Bundle(w3818, w3818, w3818, w3818, w3818, w3818) -> (w3817:cluster{dbl, dbl, dbl, dbl, dbl, dbl})  [unwired: 1 in]
                      }
                      frame True {
                        # "test on"
                        n2172 = local read "AI data 0"() -> (w3826:waveform(dbl)[])
                        n2173 = local read "AI data 1"() -> (w3825:waveform(dbl)[])
                        n2174 = local read "AI data 2"() -> (w3822:waveform(dbl)[])
                        n2175 = local read "AI Error"() -> (w3824:errorcluster[])
                        n2176 = call "sub vi - Read Analog All v9.5.vi"("data 0"=w3826, "data 1"=w3825, "data 2"=w3822, "AI Error"=w3824) -> ("array GRAPH"=w3834:dynamicdata[], "LAB01"=w3833:T31, "LAB02"=w3832:T32, "LAB03"=w3831:T33, "LAB04"=w3830:T34, "deg C"=w3828:dbl, "USB Error"=w3827:bool[], "LAB05"=w3829:T35)  [unwired: 4 in]
                        n2177 = local read "AI loop time"() -> (w3823:dbl)
                      }
                    }
                  }
                  frame True {
                    # "simulate"
                    n2178 = local read "ON amps"() -> (w3838:dbl)
                    n2179 = local read "OFF amps"() -> (w3839:dbl)
                    n2180 = local read "VOLTS"() -> (w3842:dbl)
                    n2181 = local read "PF"() -> (w3841:dbl)
                    n2182 = Select(t=w3838, s=w3844, f=w3839) -> (s? t:f=w3843:dbl)
                    n2183 = Bundle("OFF amps"=w3843, "VOLTS"=w3842, "PF"=w3841, "OFF amps"=w3843, "VOLTS"=w3842, "PF"=w3841) -> (w3840:T36)  [unwired: 1 in]
                  }
                }
                n2184 = local read "DAQ Simulate"() -> (w3798:bool)
                n2185 = stacked-sequence {
                  seq-local: [w3848 _ _ _ _ _ _ _] -> [_ _ _ _ _ _ _ _]
                  seq-local: [w3847 _ _ _ _ _ _ _] -> [_ _ _ _ _ _ _ _]
                  seq-local: [w3846 _ _ _ _ _ _ _] -> [_ _ _ _ _ _ _ w4071]
                  tunnel: w3805 -> [_ w3899 _ _ _ _ _ _]
                  tunnel: w3804 -> [_ _ w3932 _ _ _ _ _]
                  tunnel: w3803 -> [_ _ _ w3966 _ _ _ _]
                  tunnel: w3802 -> [_ _ _ _ w4000 _ _ _]
                  tunnel: w3801 -> [_ _ _ _ _ w4034 _ _]
                  tunnel: w3800 -> [_ _ _ _ _ _ w4068 _]
                  tunnel: w3798 -> [_ _ w3931 w3965 w3999 w4033 w4067 w4073]
                  tunnel: T15 {"1  (A) cal"=1.0, "1 (V) cal"=1.0, "1 (PF) cal"=1.0, "1 (TL) cal"=1.0, "1 (TN) cal"=1.0, "2 (A) cal"=1.0, "2 (V) cal"=1.0, "2 (PF) cal"=1.0, "2 (TL) cal"=1.0, "2 (TN) cal"=1.0} ("CAL LAB01") -> [_ _ w3930 w3964 w3998 w4032 w4066 _]
                  tunnel: w3795 -> [_ _ _ _ _ _ _ w4072]
                  tunnel: w3794 -> [w3851 _ _ _ _ _ _ _]
                  tunnel: w3792 -> [_ w3878 _ _ _ _ _ _]
                  frame #0 {
                    n2186 = Index Array(array=w3851, index=2) -> (element=w3846:bool)
                    n2187 = Index Array(array=w3851, index=1) -> (element=w3847:bool)
                    n2188 = Index Array(array=w3851, index=0) -> (element=w3848:bool)
                    n2189 = local write "Error USB #2"(w3846) -> ()
                    n2190 = local write "Error USB #0"(w3848) -> ()
                    n2191 = local write "Error USB #1"(w3847) -> ()
                    n2192 = stacked-sequence {
                      tunnel: w3848 -> [w3855 _ _ _]
